vi "initialise.vi"(8 "error in (no error)":errorcluster, 11 "DL090215DataCollection in":refnum<class "DataCollectionDL090215.lvclass">) -> (0 "error out":errorcluster, 3 "DL090215DataCollection out":refnum<class "DataCollectionDL090215.lvclass">)   [LabVIEW 2010, in "DataCollectionDL090215.lvclass"]
uses:
  DataCollectionDL090215.lvclass
  common/enumerations/top-level_component_type_enum.ctl
  DataCollectionDL091104Scaffold/DataCollectionDL091104Scaffold/DataCollectionDL091104Scaffold.lvclass
  DataCollectionDL090215.lvclass/DataCollectionDL090215.ctl
  common/classes/ErrorController/ErrorController/class_data.vi
  common/classes/ErrorController/ErrorController/ErrorController.lvclass
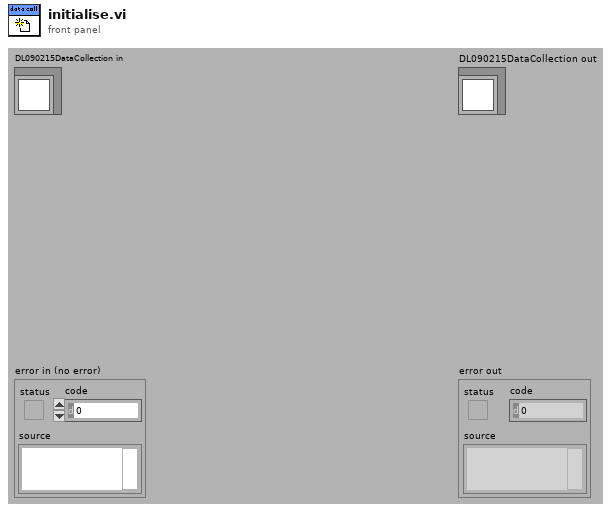
[diagram p1: front panel]
types:
  T1 = typedef "top-level_component_type_enum.ctl" = enum16{"undefined", "ImagingMode", "ScanHead", "DAQ", "ImageAssembler", "Display", "DataCollection", "Analyser", "Stimulator", "ExperimentController", "Instrument", "Stage"}
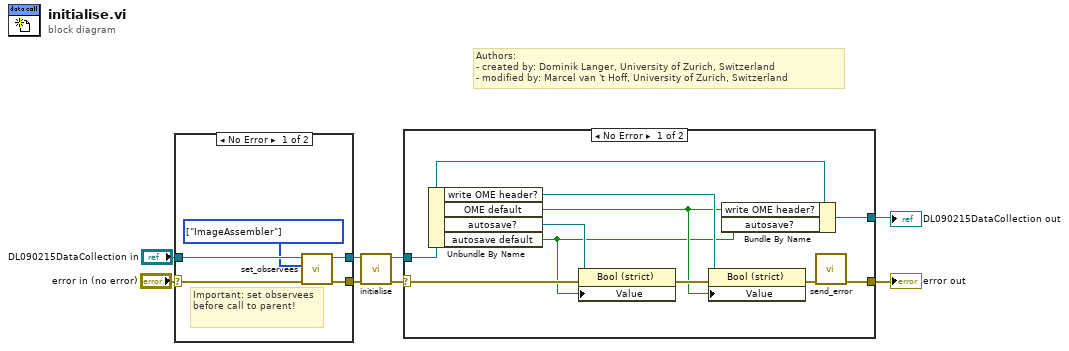
[diagram p0: block diagram]
diagram:
  # "Authors: \n- created by: Dominik Langer, University of Zurich, Switzerland\n- modified by: Marcel van 't Hoff, University of Zurich, Switzerland"
  n1 = case shown="No Error" "error in (no error)" {
    selector: "error in (no error)" -> [w13 w14]
    tunnel: [w12 w14] -> w3
    tunnel: "DL090215DataCollection in" -> [w11 w15]
    tunnel: [w10 w15] -> w1
    frame No Error {
      w9 = T1[] [enum."ImageAssembler"] items=["undefined", "ImagingMode", "ScanHead", "DAQ", "ImageAssembler", "Display", "DataCollection", "Analyser", "Stimulator", "ExperimentController", "Instrument", "Stage"] ("observees")
      # "Important: set observees before call to parent!"
      n2 = call-dynamic "set_observees.vi"("error in (no error)"=w13, "observees"=w9, "GenericToplevelComponent in"=w11) -> ("error out"=w12:errorcluster, "GenericToplevelComponent out"=w10:refnum<class "DataCollectionDL090215.lvclass">)  [unwired: 7 in]
    }
    frame Error {
    }
  }
  n3 = call-parent "initialise.vi"("error in (no error)"=w3, "DL090215DataCollection in"=w1) -> ("error out"=w8:errorcluster, "DL090215DataCollection out"=w7:refnum<class "DataCollectionDL090215.lvclass">)  [unwired: 8 out]
  n4 = case shown="No Error" w8 {
    selector: w8 -> [w20 w26]
    tunnel: w7 -> [w19 w27]
    tunnel: [w22 w26] -> w6
    tunnel: [w18 w27] -> w5
    frame No Error {
      n5 = Unbundle By Name(w19) -> ("write OME header?"=w23:refnum<vi>, "OME default"=w17:bool, "autosave?"=w25:refnum<vi>, "autosave default"=w16:bool)
      n6 = property class="Bool (strict)"(reference=w25, error in=w20, "Value"=w16) -> (error out=w24:errorcluster)  [unwired: 1 out]
      n7 = property class="Bool (strict)"(reference=w23, error in=w24, "Value"=w17) -> (error out=w21:errorcluster)  [unwired: 1 out]
      n8 = Bundle By Name(cluster=w19, "write OME header?"=w17, "autosave?"=w16) -> (w18:refnum<class "DataCollectionDL090215.lvclass">)
      n9 = call "send_error.vi"("error in (no error)"=w21) -> ("error out"=w22:errorcluster)  [unwired: 10 in]
    }
    frame Error {
    }
  }
  "error out" <- w6
  "DL090215DataCollection out" <- w5
